vi "Write Registers.vi"(8 "error in (no error)":errorcluster, 10 "Command List":T4, 11 "Serial Config":T6={"设备名称"="", "串口选择"="COM1", "仪器地址"=200, "通讯速率"=8, "超时时间"=0, "刷新时间"=10.0}) -> (0 "error out":errorcluster, 2 "Response List":T1, 3 "Status Code":string)   [LabVIEW 2010, in "MonitorServer.lvlib"]
uses:
  MonitorServer.lvlib
  Serial Config.ctl
  SubVIs/ModBUS Driver/Private/MBDRV_Command List.ctl
  SubVIs/ModBUS Driver/Private/MBDRV_Command Data.ctl
  SubVIs/ModBUS Driver/Private/MBDRV_Action.ctl
  SubVIs/ModBUS Driver/Private/MBDRV_Response List.ctl
  SubVIs/ModBUS Driver/Private/MBDRV_Response.ctl
  <vilib>/Instr/_visa.llb/VISA Configure Serial Port (Instr).vi
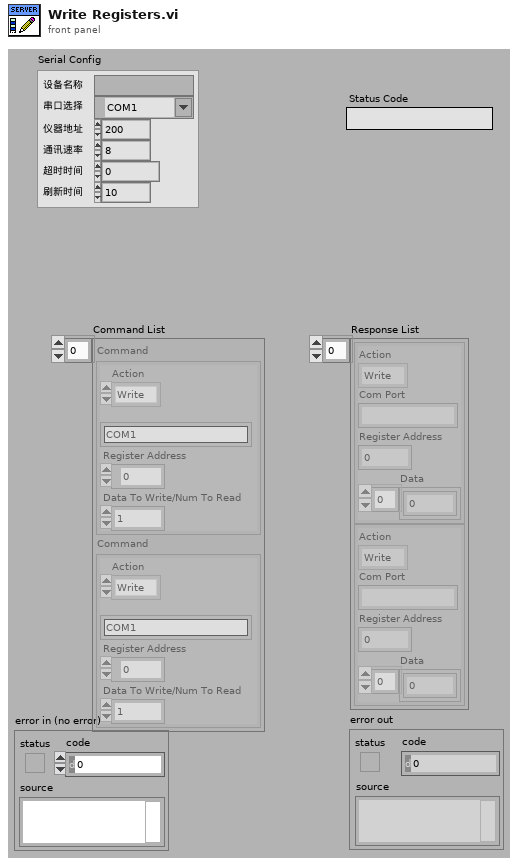
[diagram p1: front panel]
types:
  T1 = typedef "MBDRV_Response List.ctl" = T2[]
  T2 = typedef "MBDRV_Response.ctl" = cluster{"Action":T3, "Com Port":string, "Register Address":u16, "Data":i16[]}
  T3 = typedef "MBDRV_Action.ctl" = enum16{"Write", "Read"}
  T4 = typedef "MBDRV_Command List.ctl" = T5[]
  T5 = typedef "MBDRV_Command Data.ctl" = cluster{"Action":T3, "Com Port":string, "Register Address":u16, "Data To Write/Num To Read":i16}
  T6 = typedef "MonitorServer.lvlib/Serial Config.ctl" = cluster{"设备名称":string, "串口选择":refnum<visa-resource-name>, "仪器地址":u32, "通讯速率":u32, "超时时间":u32, "刷新时间":dbl}
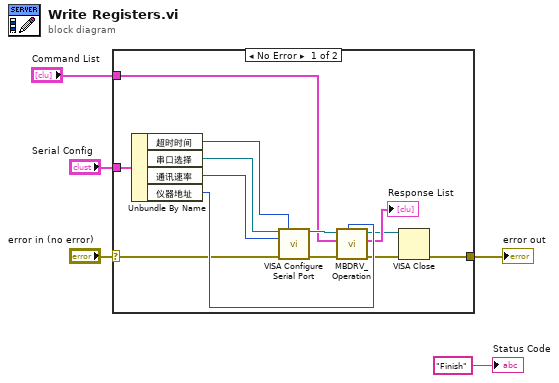
[diagram p0: block diagram]
diagram:
  n1 = case shown="No Error" "error in (no error)" {
    selector: "error in (no error)" -> [w10 w19]
    tunnel: "Serial Config" -> [w15 _]
    tunnel: [w6 w19] -> w2
    tunnel: "Command List" -> [w11 _]
    frame No Error {
      n2 = Unbundle By Name(w15) -> ("超时时间"=w16:u32, "串口选择"=w18:refnum<visa-resource-name>, "通讯速率"=w17:u32, "仪器地址"=w13:u32)
      n3 = call-poly "VISA Configure Serial Port"("VISA resource name"=w18, "timeout (10sec)"=w16, "baud rate (9600)"=w17, "error in (no error)"=w10) -> ("VISA resource name out"=w14:refnum<visa-resource-name>, "error out"=w12:errorcluster)  [unwired: 5 in, 5 out]
      n4 = call "MBDRV_Operation.vi"("Unit Address (1)"=w13, "error in (no error)"=w12, "Command List"=w11, "VISA resource name"=w14) -> ("error out"=w7:errorcluster, "Response List"=→"Response List":T1, "VISA resource name out"=w8:refnum<visa-resource-name>)  [unwired: 5 in]
      n5 = VISA Close(VISA resource name=w8, error in (no error)=w7) -> (error out=w6:errorcluster)
    }
    frame Error {
    }
  }
  "error out" <- w2
  "Status Code" <- "Finish" ("Status Code")
